vi "Add Glyph to Picture - Pixmap.vi"(4 "Mask Color (Black)":u32(colorbox), 5 "Position (0,0)":cluster{"Horizontal":i16, "Vertical":i16}, 6 "Glyph {pixmap}":u32[][](array[numeric]) format="%x", 7 "picture/image/pixmap in":picture) -> (3 "picture out":picture)   [LabVIEW 2025, in "XNode Support.lvlib"]
doc: "Adds a glyph to an image at the specified point, interpreting the \"Mask Color\" as transparent.\nThe inputs of both the image in, and the glyph can be either a Picture, an Image Cluster, or a Pixmap."
uses:
  XNode Support.lvlib
  <vilib>/picture/picture.llb/Draw True-Color Pixmap.vi
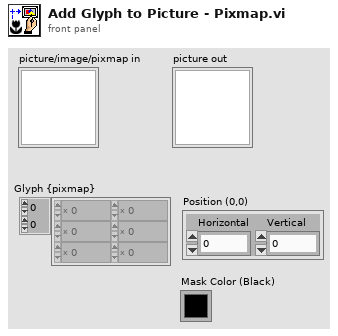
[diagram p1: front panel]
types:
  T1 = typedef "imagedata.ctl" = cluster{"image type":i32, "image depth":i32, "image":u8[], "mask":u8[], "colors":u32[], "Rectangle":cluster{"left":i16, "top":i16, "right":i16, "bottom":i16}}
  T2 = cluster{"Horizontal":i16, "Vertical":i16, "Horizontal":i16, "Vertical":i16}
  T3 = cluster{"left":i16, "top":i16, "right":i16, "bottom":i16}
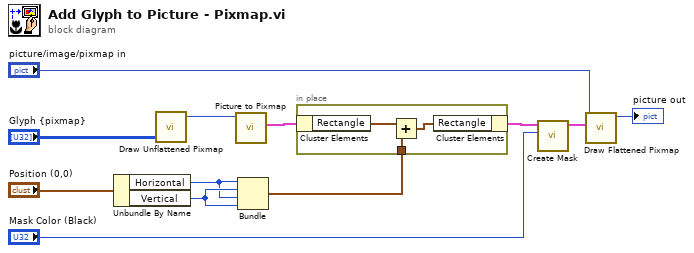
[diagram p0: block diagram]
diagram:
  n1 = Unbundle By Name("Position (0,0)") -> ("Horizontal"=w2:i16, "Vertical"=w8:i16)
  n2 = call-poly <vilib>:"Draw Unflattened Pixmap.vi"("data (RGB format)"="Glyph {pixmap}") -> ("new picture"=w1:picture)  [unwired: 8 in]
  n3 = call <vilib>:"Picture to Pixmap.vi"("picture"=w1) -> ("image data"=w4:T1)  [unwired: 9 in, 1 out]
  n4 = Bundle("Horizontal"=w2, "Vertical"=w8, "Horizontal"=w2, "Vertical"=w8) -> (w6:T2)  [unwired: 1 in]
  n5 = in-place {
    in-place-border: w6 -> [w13]
    n6 = in-place-cluster #1(w4) -> ("Rectangle"=w15:T3)
    n7 = Add(x=w15, y=w13) -> (x+y=w14:cluster{i16, i16, i16, i16})
    n8 = in-place-cluster #1("Rectangle"=w14) -> (w12:T1)
  }
  n9 = call <vilib>:"Create Mask.vi"("Mask Color (Black)"="Mask Color (Black)", "image data"=w12) -> ("image data"=w10:T1)  [unwired: 9 in]
  n10 = call <vilib>:"Draw Flattened Pixmap.vi"("image data"=w10, "picture"="picture/image/pixmap in") -> ("new picture"=→"picture out":picture)  [unwired: 7 in]
